vi "MGI Cross Product SGL.vi"(1 "B[]":sgl[](array[numeric]) format="%.2f", 2 "A[]":sgl[](array[numeric]) format="%.2f") -> (0 "AxB[]":sgl[](array[numeric]) format="%.2f")   [LabVIEW 2016]
doc: "Calculate the cross product of two 3-dimensional vectors in cartesian coordinates.\n\nAuthored by David A. Moore\nsupport@mooregoodideas.com\nwww.mooregoodideas.com\n\nCopyright (c) 2010, Moore Good Ideas, Inc.\n\nAll rights reserved.\n\nRedistribution and use in source and binary forms, with or without modification, are permitted provided that the following conditions are met:\n\n * Redistributions of source code must retain the above copyright notice, this list of conditions and the following disclaimer.\n * Redistributions in binary form must reproduce the above copyright notice, this list of conditions and the following disclaimer in the documentation and/or other materials provided with the distribution.\n * Neither the name of Moore Good Ideas, Inc. nor the names of its contributors may be used to endorse or promote products derived from this software without specific prior written permission.\n\nTHIS SOFTWARE IS PROVIDED BY THE COPYRIGHT HOLDERS AND CONTRIBUTORS \"AS IS\" AND ANY EXPRESS OR IMPLIED WARRANTIES, INCLUDING, BUT NOT LIMITED TO, THE IMPLIED WARRANTIES OF MERCHANTABILITY AND FITNESS FOR A PARTICULAR PURPOSE ARE DISCLAIMED. IN NO EVENT SHALL THE COPYRIGHT OWNER OR CONTRIBUTORS BE LIABLE FOR ANY DIRECT, INDIRECT, INCIDENTAL, SPECIAL, EXEMPLARY, OR CONSEQUENTIAL DAMAGES (INCLUDING, BUT NOT LIMITED TO, PROCUREMENT OF SUBSTITUTE GOODS OR SERVICES; LOSS OF USE, DATA, OR PROFITS; OR BUSINESS INTERRUPTION) HOWEVER CAUSED AND ON ANY THEORY OF LIABILITY, WHETHER IN CONTRACT, STRICT LIABILITY, OR TORT (INCLUDING NEGLIGENCE OR OTHERWISE) ARISING IN ANY WAY OUT OF THE USE OF THIS SOFTWARE, EVEN IF ADVISED OF THE POSSIBILITY OF SUCH DAMAGE."
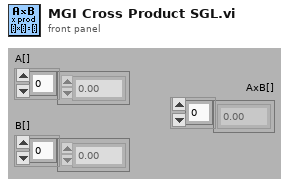
[diagram p1: front panel]
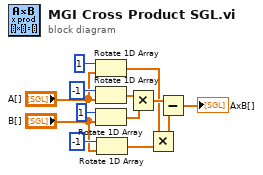
[diagram p0: block diagram]
diagram:
  n1 = Rotate 1D Array(1:"A[]", 2:1 ("n")) -> (0:w9:sgl[])
  n2 = Rotate 1D Array(1:"A[]", 2:-1 ("n")) -> (0:w7:sgl[])
  n3 = Rotate 1D Array(1:"B[]", 2:1 ("n")) -> (0:w8:sgl[])
  n4 = Rotate 1D Array(1:"B[]", 2:-1 ("n")) -> (0:w10:sgl[])
  n5 = Multiply(x=w7, y=w8) -> (x*y=w12:sgl[])
  n6 = Multiply(x=w9, y=w10) -> (x*y=w11:sgl[])
  n7 = Subtract(x=w12, y=w11) -> (x-y=→"AxB[]":sgl[])
